vi "Initialize.vi"(0 "eye scan single point":refnum<class "niHighSpeedSerial Eye Scan Single Point v1 Host.lvclass">, 5 "prescale":u8, 7 "equalization mode":T2, 9 "rx internal data width":T1=enum."32 Bit", 11 "error in":errorcluster) -> (4 "eye scan single point out":refnum<class "niHighSpeedSerial Eye Scan Single Point v1 Host.lvclass">, 15 "error out":errorcluster)   [LabVIEW 2015, in "niHighSpeedSerial Eye Scan Single Point v1 Host.lvclass"]
doc: "Configures the hardware and prepares it to be ready for Eye Scan to begin.\n\n<B>Input Parameters</B>\n\n<B>eye scan single point</B> takes in a reference to your session from the previous VI.\n\n<B>prescale</B> controls scaling of the sample count in order to keep the sample count and error count within reasonable precision.\n\n<B>equalization mode</B> indicates the Equalization Mode that the lane is using.\nenum values: DFE,LPM\n\n<B>receiver data width</B> is the data width (in bits) of the receiver lane.\nenum values: 16 Bit,20 Bit,32 Bit,40 Bit\n\n<B>error in</B> describes error conditions that occur before this node runs. This input provides standard 'error in' functionality.\n\n<B>Output Parameters</B>\n\n<B>eye scan single point out</B> passes a reference to your session to the next VI.\n\n<B>error out</B> contains error information. This output provides standard 'error out' functionality."
uses:
  <instrlib>/niHighSpeedSerial/Eye Scan/v1/Host/Impl/Single Point/niHighSpeedSerial Eye Scan Single Point v1 Host.lvclass
  <instrlib>/niHighSpeedSerial/Eye Scan/v1/Host/Common/Public/Equalization Mode.ctl
  <instrlib>/niHighSpeedSerial/Eye Scan/v1/Host/Common/Public/Data Width.ctl
  <instrlib>/niHighSpeedSerial/Eye Scan/v1/Host/Impl/Single Point/niHighSpeedSerial Eye Scan Single Point v1 Host.lvclass/niHighSpeedSerial Eye Scan Single Point v1 Host.ctl
  <instrlib>/niHighSpeedSerial/Eye Scan/v1/Host/Impl/Single Point/Private/Channel Measure State.ctl
  <vilib>/Utility/error.llb/Error Cluster From Error Code.vi
  <vilib>/ErrorRing/Error Ring.xnode
  <instrlib>/niHighSpeedSerial/Eye Scan/v1/Host/Common/niHighSpeedSerial Eye Scan Common v1 Host.lvlib
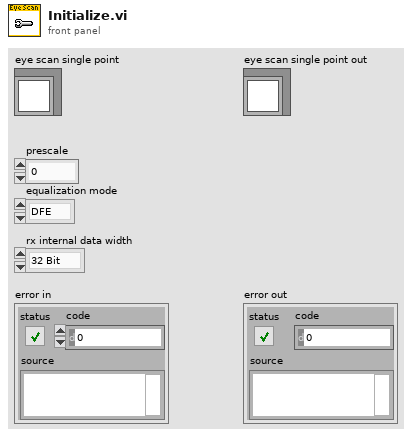
[diagram p1: front panel]
types:
  T1 = typedef "niHighSpeedSerial Eye Scan Common v1 Host.lvlib/Data Width.ctl" = enum16{"16 Bit", "20 Bit", "32 Bit", "40 Bit"}
  T2 = typedef "niHighSpeedSerial Eye Scan Common v1 Host.lvlib/Equalization Mode.ctl" = enum16{"DFE", "LPM"}
  T3 = typedef "niHighSpeedSerial Eye Scan Single Point v1 Host.lvclass/Channel Measure State.ctl" = enum16{"Uninitialized", "Initialized", "Ready", "Request", "Wait", "Read", "Process", "Finished"}
  T4 = typedef "niHighSpeedSerial Eye Scan Single Point v1 Host.lvclass/Private Data.ctl" = cluster{"GTX2_CHANNEL register map":refnum<class "GTX2_CHANNEL Register Map.lvclass">, "instruction target":refnum<class "niInstr Instruction Target v1 Host.lvclass">, "channel measure state":T3, "in DFE mode?":bool, "prescale":u8, "rx internal data width":T1, "active point":T5, "ut sign":T6, "positive counts":T7, "negative counts":T7}
  T5 = typedef "niHighSpeedSerial Eye Scan Common v1 Host.lvlib/Point Offsets.ctl" = cluster{"horizontal offset":i16, "vertical offset":i8}
  T6 = typedef "GTX2_CHANNEL v1 Host.lvlib/ESVertOffsetSign.ctl" = enum8{"Positive", "Negative"}
  T7 = typedef "niHighSpeedSerial Eye Scan Single Point v1 Host.lvclass/Counts.ctl" = cluster{"sample count":u64, "error count":u16}
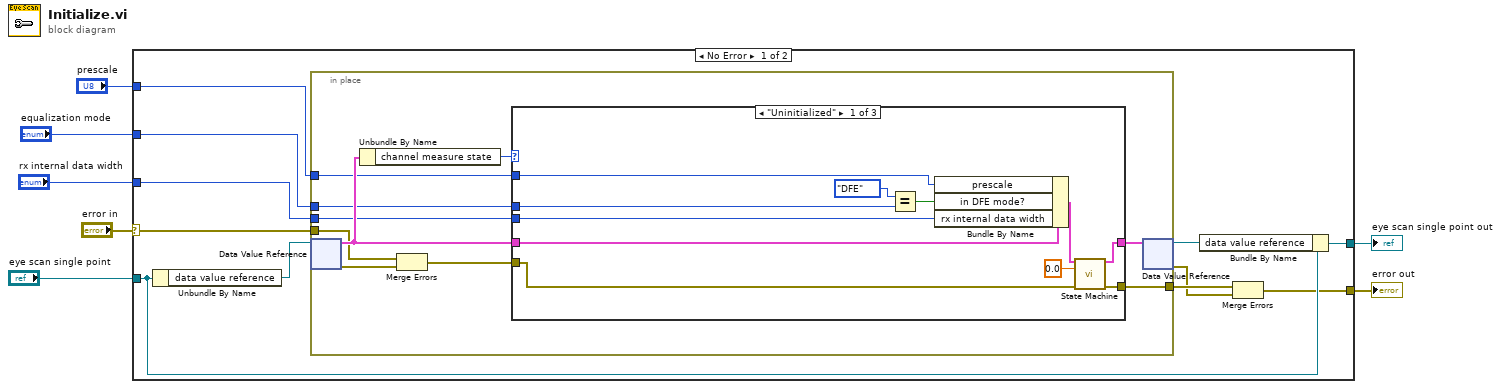
[diagram p0: block diagram]
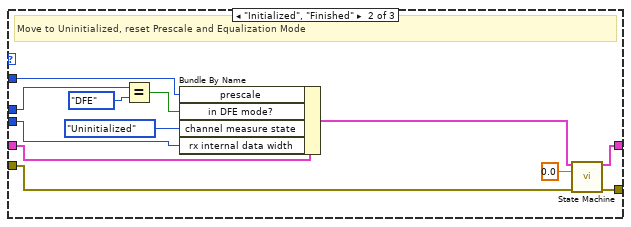
[diagram p2: hidden frame]
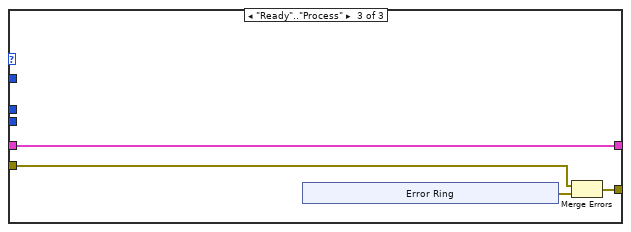
[diagram p3: hidden frame]
diagram:
  n1 = case shown="No Error" "error in" {
    selector: "error in" -> [w14 w61]
    tunnel: [w12 w61] -> w6
    tunnel: [w17 w60] -> w5
    tunnel: "eye scan single point" -> [w18 w60]
    tunnel: "equalization mode" -> [w10 _]
    tunnel: "prescale" -> [w9 _]
    tunnel: "rx internal data width" -> [w8 _]
    frame No Error {
      n2 = Unbundle By Name(w18) -> ("data value reference"=w16:refnum<data-value>)
      n3 = in-place {
        in-place-border: w14 -> [w27]
        in-place-border: [w24] -> w13
        in-place-border: w10 -> [w21]
        in-place-border: w9 -> [w20]
        in-place-border: w8 -> [w19]
        n4 = in-place-dvr #1(w16) -> (w28:T4, w26:errorcluster)
        n5 = Unbundle By Name(w28) -> ("channel measure state"=w22:T3)
        n6 = Merge Errors(w27, w26) -> (w25:errorcluster)
        n7 = case shown="\"Uninitialized\"" w22 {
          tunnel: w28 -> [w31 w51 w53]
          tunnel: w25 -> [w39 w45 w55]
          tunnel: [w38 w43 w54] -> w24
          tunnel: [w37 w44 w53] -> w23
          tunnel: w21 -> [w34 w49 _]
          tunnel: w20 -> [w32 w50 _]
          tunnel: w19 -> [w29 w40 _]
          frame "Uninitialized" {
            n8 = Equal?(x=Equalization_Mode."DFE" ("y"), y=w34) -> (x = y?=w33:bool)
            n9 = Bundle By Name(cluster=w31, "prescale"=w32, "in DFE mode?"=w33, "rx internal data width"=w29) -> (w30:T4)
            n10 = call <instrlib>:"State Machine.vi"("private data"=w30, "timeout (100 ms)"=0.0 ("Timeout (100 ms)"), "error in"=w39) -> ("private data out"=w37:T4, "error out"=w38:errorcluster)  [unwired: 6 in, 5 out]
          }
          frame "Initialized", "Finished" {
            # "Move to Uninitialized, reset Prescale and Equalization Mode"
            n11 = Equal?(x=w49, y=Equalization_Mode."DFE") -> (x = y?=w48:bool)
            n12 = Bundle By Name(cluster=w51, "prescale"=w50, "in DFE mode?"=w48, "channel measure state"=Channel_Measure_State."Uninitialized" ("Channel Measure State"), "rx internal data width"=w40) -> (w46:T4)
            n13 = call <instrlib>:"State Machine.vi"("private data"=w46, "timeout (100 ms)"=0.0 ("Timeout (100 ms)"), "error in"=w45) -> ("private data out"=w44:T4, "error out"=w43:errorcluster)  [unwired: 6 in, 5 out]
          }
          frame "Ready".."Process" {
            n14 = xnode "Error Ring"() -> ("error out"=w52:errorcluster)
            n15 = Merge Errors(w55, w52) -> (w54:errorcluster)
          }
        }
        n16 = in-place-dvr #1(w23) -> (w15:refnum<data-value>, w11:errorcluster)
      }
      n17 = Bundle By Name(cluster=w18, "data value reference"=w15) -> (w17:refnum<class "niHighSpeedSerial Eye Scan Single Point v1 Host.lvclass">)
      n18 = Merge Errors(w13, w11) -> (w12:errorcluster)
    }
    frame Error {
    }
  }
  "eye scan single point out" <- w5
  "error out" <- w6
